vi "Continuous Volume Demo.vi"() -> ()   [LabVIEW 2012]
uses:
  LabVIEW/user.lib/SpectralRadar.llb/Data Analyzation Selection.ctl
  LabVIEW/user.lib/SpectralRadar.llb/Device Camera Preset Selection.ctl
  LabVIEW/user.lib/SpectralRadar.llb/Processing Flag Selection.ctl
  LabVIEW/user.lib/SpectralRadar.llb/ScanPattern_ApodizationType.ctl
  LabVIEW/user.lib/SpectralRadar.llb/ScanPattern_AcquisitionOrder.ctl
  LabVIEW/user.lib/SpectralRadar.llb/Normal Direction Selection.ctl
  LabVIEW/user.lib/SpectralRadar.llb/set Apodized Spectrum Output.vi
  LabVIEW/user.lib/SpectralRadar.llb/set Scan Output.vi
  LabVIEW/user.lib/SpectralRadar.llb/display Data 2D.vi
  LabVIEW/user.lib/SpectralRadar.llb/OCT Device.lvclass
  LabVIEW/user.lib/SpectralRadar.llb/Probe.lvclass
  LabVIEW/user.lib/SpectralRadar.llb/Processing.lvclass
  LabVIEW/user.lib/SpectralRadar.llb/Raw Data.lvclass
  LabVIEW/user.lib/SpectralRadar.llb/Data.lvclass
  LabVIEW/user.lib/SpectralRadar.llb/Scan Pattern.lvclass
panel:
  in  "Slice vs. Process":bool
  in  "Data Analyzation Selection":T1
  out "B-Scan Data":dbl[][](graph)
  in  "Index":i32(slide) min=0 max=1023 step=1 scale=0.0..1023.0
  in  "stop":bool
  out "En-Face Data":dbl[][](graph)
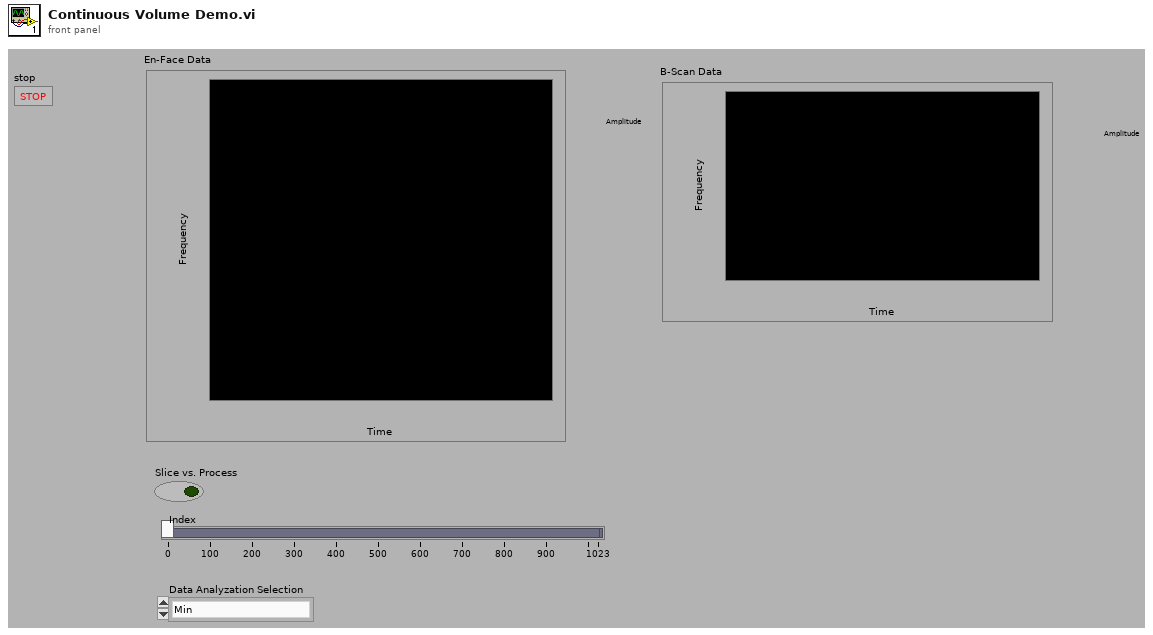
[diagram p1: front panel]
types:
  T1 = typedef "Data.lvclass/Data Analyzation Selection.ctl" = enum16{"Min", "Mean", "Max"}
  T2 = typedef "Scan Pattern.lvclass/ScanPattern_AcquisitionOrder.ctl" = u16
  T3 = typedef "Scan Pattern.lvclass/ScanPattern_ApodizationType.ctl" = u16
  T4 = typedef "Processing.lvclass/Processing Flag Selection.ctl" = enum16{"Use Offset Errors", "Remove DC Spectrum", "Remove Advanced DC Spectrum", "Use Apodization", "Use Scan For Apodization", "Filter Undersampled Signals", "Use Dispersion Compensation", "Use Dechirp", "Use Extended Adjust", "Full Range Output", "Filter DC", "Autocorrelation Compensation", "DEFR", "Only Windowing", "Remove Fixed Pattern", "Calculate Saturation"}
  T5 = typedef "OCT Device.lvclass/Device Camera Preset Selection.ctl" = enum16{"Default", "Preset 1", "Preset 2", "Preset 3"}
  T6 = enum16{"Asynchronous Continuous", "Asynchronous Finite", "Synchronous"}
  T7 = typedef "Data.lvclass/Normal Direction Selection.ctl" = enum16{"Direction 1", "Direction 2", "Direction 3"}
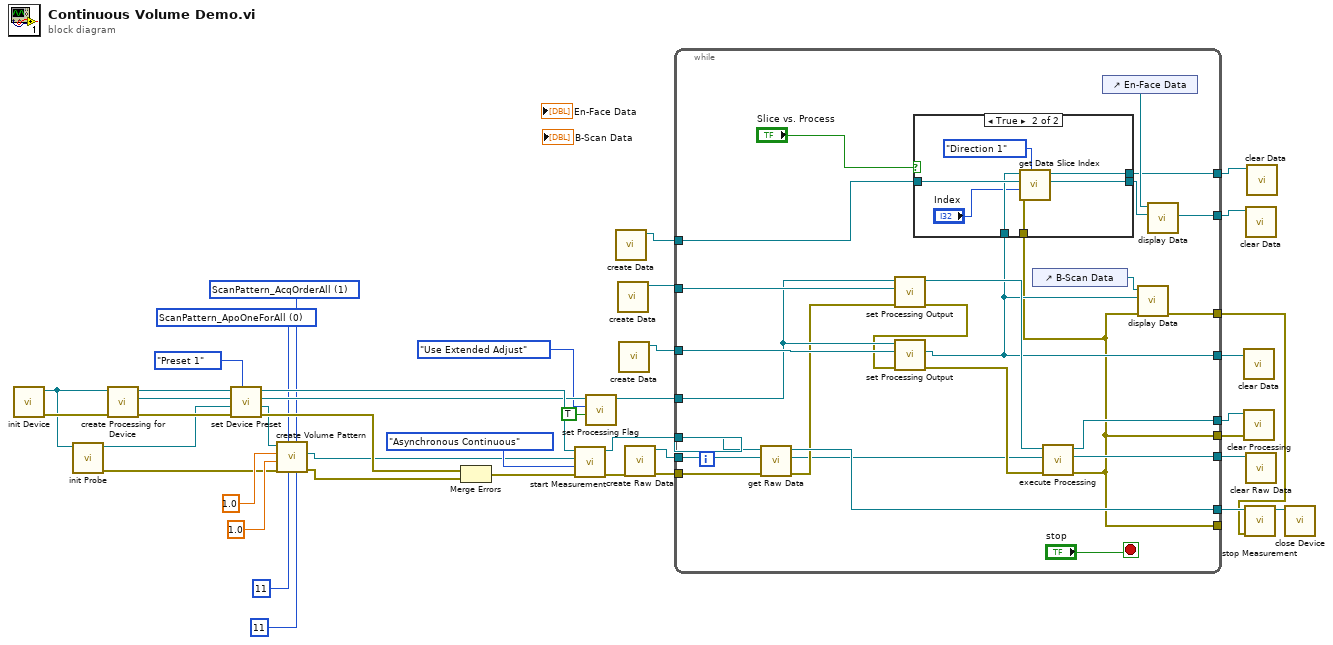
[diagram p0: block diagram]
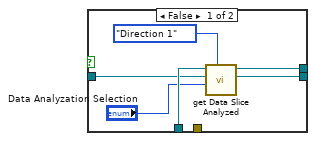
[diagram p2: hidden frame]
diagram:
  w1 = T2 1 items=["ScanPattern_AcqOrderFrameByFrame", "ScanPattern_AcqOrderAll"] ("Acquisition order")
  w2 = T3 0 items=["ScanPattern_ApoOneForAll", "ScanPattern_ApoEachBScan"] ("Apodization type")
  n1 = call "init Device.vi"() -> ("error out"=w40:errorcluster, "OCTDevice"=w32:refnum<class "OCT Device.lvclass">)  [unwired: 6 in]
  n2 = call "init Probe.vi"("OCT Device"=w32) -> ("error out"=w18:errorcluster, "GalvoControl"=w27:refnum<class "Probe.lvclass">)  [unwired: 5 in]
  n3 = call "create Processing for Device.vi"("error in (no error)"=w40, "OCTDevice"=w32) -> ("error out"=w37:errorcluster, "Processing"=w25:refnum<class "Processing.lvclass">, "OCTDevice"=w28:refnum<class "OCT Device.lvclass">)  [unwired: 3 in]
  n4 = call "set Device Preset.vi"("Numeric"=Device_Camera_Preset_Selection."Preset 1" ("Device Camera Preset Selection"), "Probe"=w27, "Processing"=w25, "OCTDevice"=w28) -> ("Probe 2"=w23:refnum<class "Probe.lvclass">, "Processing"=w15:refnum<class "Processing.lvclass">, "OCTDevice out"=w26:refnum<class "OCT Device.lvclass">)  [unwired: 2 in, 1 out]
  n5 = call "create Volume Pattern.vi"("Size Y"=11, "Acquisition order"=w1, "Size X"=11, "Apodization type"=w2, "error in (no error)"=w18, "Range Y"=1.0, "Range X"=1.0, "Probe"=w23) -> ("error out"=w17:errorcluster, "Scan Pattern"=w16:refnum<class "Scan Pattern.lvclass">)  [unwired: 1 in, 1 out]
  n6 = Merge Errors(w37, w17) -> (w38:errorcluster)
  n7 = call "start Measurement.vi"("error in (no error)"=w38, "Acquisition Type"=T6."Asynchronous Continuous", "Scan Pattern"=w16, "OCTDevice"=w26) -> ("error out"=w35:errorcluster, "OCTDevice"=w29:refnum<class "OCT Device.lvclass">)  [unwired: 1 in, 1 out]
  n8 = call "set Processing Flag.vi"("Flag"=TRUE, "Processing Flag Selection"=Processing_Flag_Selection."Use Extended Adjust", "Processing"=w15) -> ("Processing"=w14:refnum<class "Processing.lvclass">)  [unwired: 3 in, 1 out]
  n9 = call "create Data.vi"() -> ("Data"=w3:refnum<class "Data.lvclass">)  [unwired: 6 in, 1 out]
  n10 = call "create Data.vi"() -> ("Data"=w4:refnum<class "Data.lvclass">)  [unwired: 6 in, 1 out]
  n11 = call "create Data.vi"() -> ("Data"=w5:refnum<class "Data.lvclass">)  [unwired: 6 in, 1 out]
  n12 = call "create Raw Data.vi"("error in (no error)"=w35) -> ("error out"=w34:errorcluster, "Raw Data"=w36:refnum<class "Raw Data.lvclass">)  [unwired: 5 in]
  n13 = while {
    tunnel: w36 -> [w64]
    tunnel: w29 -> [w65]
    tunnel: w34 -> [w63]
    tunnel: w14 -> [w60]
    tunnel: w5 -> [w62]
    tunnel: w4 -> [w61]
    tunnel: [w55] -> w33
    tunnel: [w54] -> w10
    tunnel: [w44] -> w8
    tunnel: [w53] -> w31
    tunnel: [w43] -> w9
    tunnel: [w43] -> _
    tunnel: w3 -> [w49]
    tunnel: [w48] -> w7
    tunnel: [w46] -> w6
    tunnel: [w41] -> w11
    stop <- "stop" stop-if-true
    n14 = call "get Raw Data.vi"("error in (no error)"=w63, "RawData in"=w64, "OCTDevice in"=w65) -> ("error out"=w52:errorcluster, "RawData out"=w50:refnum<class "Raw Data.lvclass">, "OCTDevice out"=w53:refnum<class "OCT Device.lvclass">)  [unwired: 2 in]
    n15 = call-poly "set Processing Output.vi"("error in (no error)"=w52, "Data"=w61, "Processing"=w60) -> ("error out"=w58:errorcluster, "Processing"=w59:refnum<class "Processing.lvclass">)  [unwired: 2 in, 1 out]
    n16 = call-poly "set Processing Output.vi"("error in (no error)"=w58, "Data"=w62, "Processing"=w60) -> ("error out"=w57:errorcluster, "Data"=w44:refnum<class "Data.lvclass">)  [unwired: 2 in, 1 out]
    n17 = control-ref of="B-Scan Data"() -> (w45:refnum<vi>)
    n18 = call "execute Processing.vi"("error in (no error)"=w57, "Raw Data"=w50, "Processing"=w59) -> ("error out"=w43:errorcluster, "Raw Data"=w55:refnum<class "Raw Data.lvclass">, "Processing"=w54:refnum<class "Processing.lvclass">)  [unwired: 2 in]
    n19 = case shown="True" "Slice vs. Process" {
      tunnel: w49 -> [w70 w78]
      tunnel: [w66 w76] -> w47
      tunnel: [w67 w75] -> w46
      tunnel: w44 -> [w71 w74]
      tunnel: w43 -> [_ w73]
      frame False {
        n20 = call "get Data Slice Analyzed.vi"("Normal Direction"=Normal_Direction_Selection."Direction 1", "Data Analyzation Selection"="Data Analyzation Selection", "Slice"=w70, "Data"=w71) -> ("Slice"=w66:refnum<class "Data.lvclass">, "Data"=w67:refnum<class "Data.lvclass">)  [unwired: 3 in, 1 out]
      }
      frame True {
        n21 = call "get Data Slice Index.vi"("Normal Direction"=Normal_Direction_Selection."Direction 1", "error in (no error)"=w73, "Index"="Index", "Slice"=w78, "Data"=w74) -> ("Slice"=w76:refnum<class "Data.lvclass">, "Data"=w75:refnum<class "Data.lvclass">)  [unwired: 2 in, 1 out]
      }
    }
    n22 = control-ref of="En-Face Data"() -> (w56:refnum<vi>)
    n23 = call-poly "display Data.vi"("error in (no error)"=w43, "Data in"=w44, "IntGraph Refnum"=w45) -> ("error out"=w41:errorcluster)  [unwired: 2 in, 2 out]
    n24 = call-poly "display Data.vi"("Data in"=w47, "IntGraph Refnum"=w56) -> ("Data out"=w48:refnum<class "Data.lvclass">)  [unwired: 3 in, 2 out]
  }
  n25 = call "clear Data.vi"("Data"=w8) -> ()  [unwired: 6 in, 1 out]
  n26 = call "clear Processing.vi"("error in (no error)"=w9, "Processing"=w10) -> ()  [unwired: 5 in, 1 out]
  n27 = call "stop Measurement.vi"("error in (no error)"=w11, "OCTDevice"=w31) -> ("OCTDevice"=w30:refnum<class "OCT Device.lvclass">)  [unwired: 4 in, 1 out]
  n28 = call "clear Data.vi"("Data"=w7) -> ()  [unwired: 6 in, 1 out]
  n29 = call "clear Raw Data.vi"("Raw Data"=w33) -> ()  [unwired: 6 in, 1 out]
  n30 = call "clear Data.vi"("Data"=w6) -> ()  [unwired: 6 in, 1 out]
  n31 = call "close Device.vi"("OCTDevice"=w30) -> ()  [unwired: 6 in, 1 out]
